vi "USB XYZ Stage Reference.vi"() -> ()   [LabVIEW 2018]
panel:
  in  "XYZ STAGE USB REFERENCE":i32
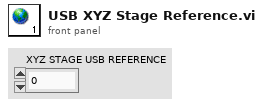
[diagram p1: front panel]
diagram:
